vi "CutImageBorder.vi"(8 "削除枠幅":cluster{"左":i16, "上":i16, "右":i16, "下":i16}, 11 "元画像":T1 caption="画像データ") -> (3 "切抜き画像":T1 caption="部分画像")   [LabVIEW 2014]
uses:
  <vilib>/picture/picture.llb/imagedata.ctl
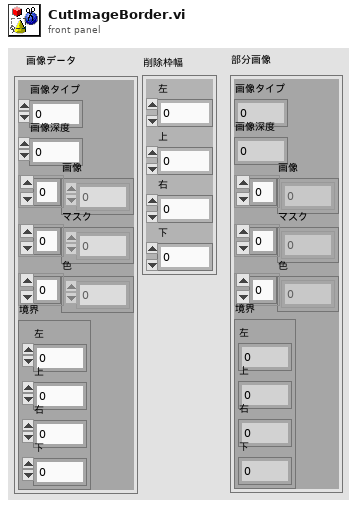
[diagram p1: front panel]
types:
  T1 = typedef "imagedata.ctl" = cluster{"image type":i32, "image depth":i32, "image":u8[], "mask":u8[], "colors":u32[], "Rectangle":cluster{"left":i16, "top":i16, "right":i16, "bottom":i16}}
  T2 = cluster{"left":i16, "top":i16, "right":i16, "bottom":i16}
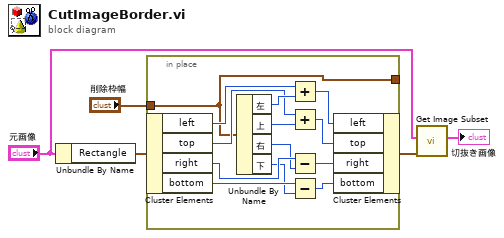
[diagram p0: block diagram]
diagram:
  n1 = Unbundle By Name("元画像") -> ("Rectangle"=w3:T2)
  n2 = in-place {
    in-place-border: [w13] -> _
    in-place-border: "削除枠幅" -> [w13]
    n3 = in-place-cluster #1(w3) -> ("left"=w16:i16, "top"=w15:i16, "right"=w11:i16, "bottom"=w8:i16)
    n4 = Unbundle By Name(w13) -> ("左"=w18:i16, "上"=w17:i16, "右"=w10:i16, "下"=w7:i16)
    n5 = Add(x=w16, y=w18) -> (x+y=w14:i16)
    n6 = Add(x=w15, y=w17) -> (x+y=w12:i16)
    n7 = Subtract(x=w11, y=w10) -> (x-y=w9:i16)
    n8 = Subtract(x=w8, y=w7) -> (x-y=w6:i16)
    n9 = in-place-cluster #1("left"=w14, "top"=w12, "right"=w9, "bottom"=w6) -> (w2:T2)
  }
  n10 = call <vilib>:"Get Image Subset.vi"("subset rect"=w2, "image data"="元画像") -> ("image subset"=→"切抜き画像":T1)  [unwired: 4 in, 1 out]
